vi "SingleExecution.vi"() -> ()   [LabVIEW 2012]
panel:
  in  "Frame Index (0)":u32
  in  "Connection Mode":enum32{"INIT_FILE", "INIT_LIVE"}(radio)
  in  "USB Device Name":string="AC12345"
  in  "Path to Record":path=path "D:/R&D-2013-06-19-14-07-16-824.ltl"
  # "This VI implements a very simple single execution example.\nBefore execution, fill either the path to record or the USB device name.\nFrame index is required when in file mode only.\nThen select the appropriate connection mode.\nFinally open FanGraph.vi to see its update and run once SingleExecution.vi."
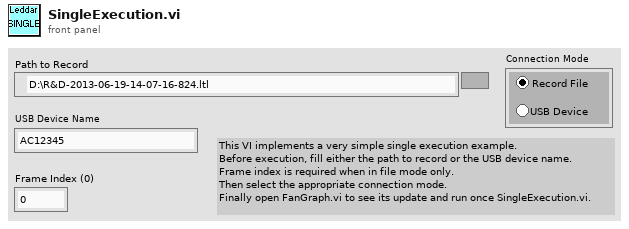
[diagram p1: front panel]
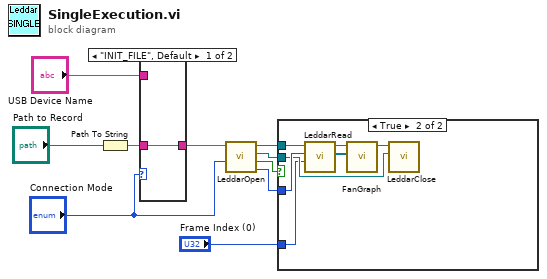
[diagram p0: block diagram]
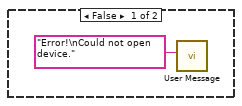
[diagram p2: hidden frame]
diagram:
  n1 = Path To String(path="Path to Record") -> (string=w8:string)
  n2 = case shown="\"INIT_FILE\", Default" "Connection Mode" {
    tunnel: "USB Device Name" -> [_ w12]
    tunnel: w8 -> [w11 _]
    tunnel: [w11 w12] -> w7
    frame "INIT_FILE", Default {
    }
    frame "INIT_LIVE" {
    }
  }
  n3 = call "LeddarOpen.vi"("Connection Mode"="Connection Mode", "File path, USB name"=w7) -> ("Connection Mode Out"=w5:enum32{"INIT_FILE", "INIT_LIVE"}, "Success"=w1:bool, "Event Callback"=w3:refnum<k27>, "DeviceControl"=w4:refnum<k24>)  [unwired: 6 in]
  n4 = case shown="True" w1 {
    tunnel: w5 -> [_ w20]
    tunnel: w4 -> [_ w19]
    tunnel: w3 -> [_ w18]
    tunnel: "Frame Index (0)" -> [_ w14]
    frame False {
      n5 = call "User Message"("Message"="Error!\nCould not open device.") -> ()  [unwired: 9 in, 2 out]
    }
    frame True {
      n6 = call "LeddarRead.vi"("Frame Index"=w14, "Connection Mode"=w20, "DeviceControl"=w19) -> ("Detections Array"=w17:refnum<k24>[], "DeviceControl Out"=w16:refnum<k24>)  [unwired: 6 in, 1 out]
      n7 = call "FanGraph.vi"("DeviceControl"=w16, "Detections"=w17) -> ("DeviceControl Out"=w15:refnum<k24>)  [unwired: 8 in]
      n8 = call "LeddarClose.vi"("Event Callback"=w18, "DeviceControl"=w15) -> ()  [unwired: 10 in]
    }
  }
